vi "DateTabTimeString.vi"(2 "Seconds?":bool) -> (0 "Date/Time String":string)   [LabVIEW 2013]
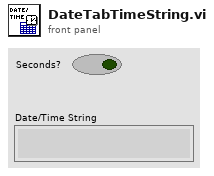
[diagram p1: front panel]
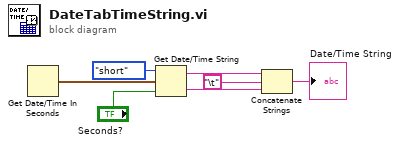
[diagram p0: block diagram]
diagram:
  n1 = Get Date/Time In Seconds() -> (seconds since 1Jan1904=w7:timestamp)
  n2 = Get Date/Time String(date format (0)=enum16{"short", "long", "abbreviated"}."short", seconds (now)=w7, want seconds? (F)="Seconds?") -> (date string=w5:string, time string=w3:string)
  n3 = Concatenate Strings(w5, "\t", w3) -> (→"Date/Time String":string)
